vi "Calculate Analog and Digital Channel Values.vi"(9 "Execute Sequence":bool=TRUE, 10 "current time":timestamp, 11 "Settings in":T1) -> (0 "Digital Values to Write":bool[](array[boolean]), 1 "Analog Values to Write":dbl[](array[numeric]), 2 "Sequence State Channels to Write":dbl[](array[numeric]), 3 "Settings out":T1)   [LabVIEW 2020]
uses:
  Params.ctl
  Step Settings.ctl
  Sequencer with Output Values.lvclass
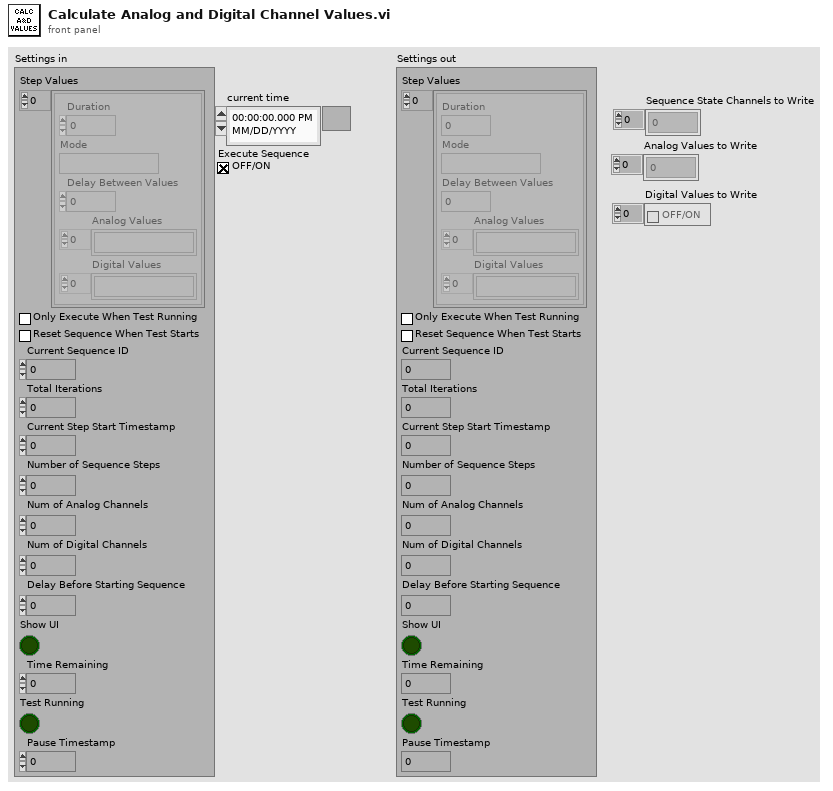
[diagram p1: front panel]
types:
  T1 = typedef "Sequencer with Output Values.lvlib/Sequencer with Output Values.lvclass/Params.ctl" = cluster{"Step Values":T2[], "Only Execute When Test Running":bool, "Reset Sequence When Test Starts":bool, "Current Sequence ID":u32, "Total Iterations":u32, "Current Step Start Timestamp":dbl, "Number of Sequence Steps":i32, "Num of Analog Channels":i32, "Num of Digital Channels":i32, "Delay Before Starting Sequence":dbl, "Show UI":bool, "Time Remaining":dbl, "Test Running":bool, "Pause Timestamp":dbl}
  T2 = typedef "Sequencer with Output Values.lvlib/Sequencer with Output Values.lvclass/Step Settings.ctl" = cluster{"Duration":dbl, "Mode":string, "Delay Between Values":dbl, "Analog Values":string[], "Digital Values":string[]}
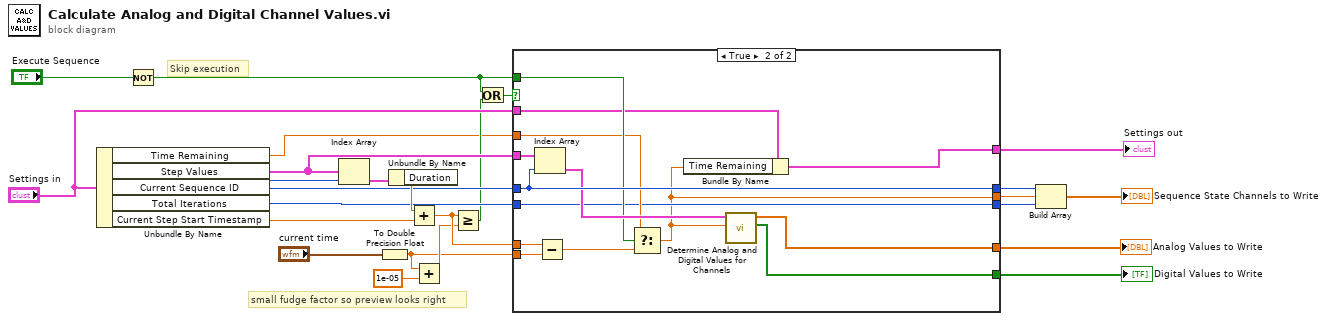
[diagram p0: block diagram]
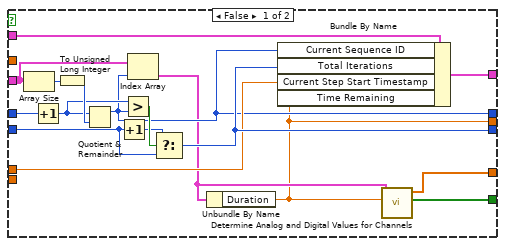
[diagram p2: hidden frame]
diagram:
  # "Skip execution"
  # "small fudge factor so preview looks right"
  n1 = Unbundle By Name("Settings in") -> ("Time Remaining"=w2:dbl, "Step Values"=w17:T2[], "Current Sequence ID"=w19:u32, "Total Iterations"=w18:u32, "Current Step Start Timestamp"=w20:dbl)
  n2 = Not(x="Execute Sequence") -> (.not. x?=w1:bool)
  n3 = Index Array(array=w17, index=w19) -> (element=w23:T2)
  n4 = To Double Precision Float(number="current time") -> (double precision float=w12:dbl)
  n5 = Unbundle By Name(w23) -> ("Duration"=w21:dbl)
  n6 = Add(x=w21, y=w20) -> (x+y=w22:dbl)
  n7 = Add(x=w12, y=1e-05) -> (x+y=w13:dbl)
  n8 = Greater Or Equal?(x=w22, y=w13) -> (x >= y?=w4:bool)
  n9 = Or(x=w1, y=w4) -> (x .or. y?=w5:bool)
  n10 = case shown="True" w5 {
    tunnel: "Settings in" -> [w36 w45]
    tunnel: w19 -> [w40 w52]
    tunnel: w17 -> [w30 w53]
    tunnel: w18 -> [w38 w44]
    tunnel: [w29 w52] -> w10
    tunnel: [w34 w44] -> w9
    tunnel: [w35 w43] -> w24
    tunnel: w22 -> [w31 w55]
    tunnel: w12 -> [_ w54]
    tunnel: [w25 w42] -> w11
    tunnel: [w28 w50] -> w8
    tunnel: [w27 w49] -> w7
    tunnel: w1 -> [_ w47]
    tunnel: w2 -> [_ w46]
    frame False {
      n11 = Array Size(array=w30) -> (size(s)=w41:i32)
      n12 = Increment(x=w40) -> (x+1=w32:u32)
      n13 = To Unsigned Long Integer(number=w41) -> (unsigned 32bit integer=w33:u32)
      n14 = Quotient & Remainder(x=w32, y=w33) -> (x-y*floor(x/y)=w29:u32)  [unwired: 1 out]
      n15 = Increment(x=w38) -> (x+1=w37:u32)
      n16 = Greater?(x=w32, y=w29) -> (0:w39:bool)
      n17 = Index Array(array=w30, index=w29) -> (element=w26:T2)
      n18 = Select(t=w37, s=w39, f=w38) -> (s? t:f=w34:u32)
      n19 = Unbundle By Name(w26) -> ("Duration"=w25:dbl)
      n20 = Bundle By Name(cluster=w36, "Current Sequence ID"=w29, "Total Iterations"=w34, "Current Step Start Timestamp"=w31, "Time Remaining"=w25) -> (w35:T1)
      n21 = call "Determine Analog and Digital Values for Channels.vi"("Remaining Time"=w25, "Step Settings"=w26) -> ("Digital Values to Write"=w27:bool[], "Analog Values to Write"=w28:dbl[])  [unwired: 8 in]
    }
    frame True {
      n22 = Index Array(array=w53, index=w52) -> (element=w51:T2)
      n23 = Subtract(x=w55, y=w54) -> (x-y=w48:dbl)
      n24 = Select(t=w46, s=w47, f=w48) -> (s? t:f=w42:dbl)
      n25 = Bundle By Name(cluster=w45, "Time Remaining"=w42) -> (w43:T1)
      n26 = call "Determine Analog and Digital Values for Channels.vi"("Remaining Time"=w42, "Step Settings"=w51) -> ("Digital Values to Write"=w49:bool[], "Analog Values to Write"=w50:dbl[])  [unwired: 8 in]
    }
  }
  "Settings out" <- w24
  "Digital Values to Write" <- w7
  "Analog Values to Write" <- w8
  n27 = Build Array(w10, w11, w9) -> (→"Sequence State Channels to Write":dbl[])
